vi "Read User Tag.vi"(8 "error in":errorcluster, 11 "MB_TCP session in":refnum<class "MB_Master_TCP.lvclass">) -> (0 "error out":errorcluster, 2 "Value":string, 3 "MB session out":refnum<class "MB_Master_TCP.lvclass">)   [LabVIEW 2024, in "Bronkhorst Flexi-Flow ModbusTCP API.lvlib"]
uses:
  Bronkhorst Flexi-Flow ModbusTCP API.lvlib
  <vilib>/Plasmionique/MB Master/MB_Master_TCP/MB_Master_TCP.lvclass
  PDU Address String Params--ring.ctl
  <vilib>/Utility/error.llb/whitespace.ctl
  <vilib>/Utility/error.llb/Trim Whitespace One-Sided.vi
  Read String Register.vi
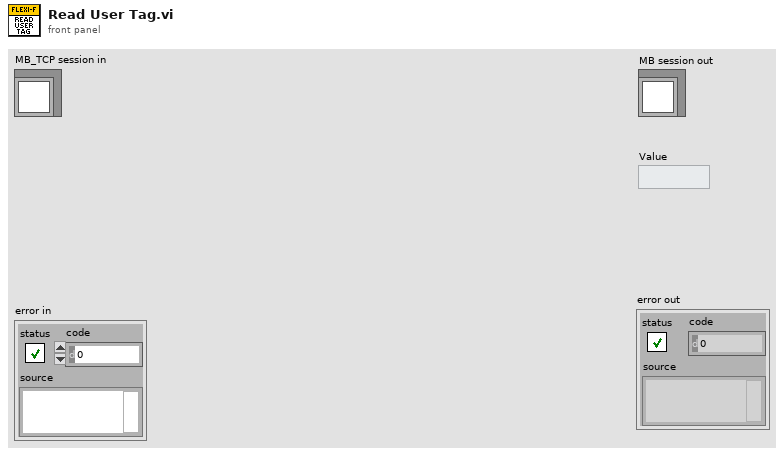
[diagram p1: front panel]
types:
  T1 = typedef "whitespace.ctl" = u16
  T2 = typedef "Bronkhorst Flexi-Flow ModbusTCP API.lvlib/PDU Address String Params--ring.ctl" = u16
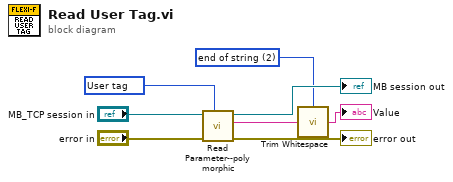
[diagram p0: block diagram]
diagram:
  w1 = T1 2 items=["both", "start of string", "end of string"] ("location (both)")
  w8 = T2 61744 items=["Fluid name"=33160, "Capacity unit"=33272, "User tag"=61744] ("PDU Address String Params")
  n1 = call-poly "Read Parameter--polymorphic.vi"("PDU Address String Params"=w8, "error in"="error in", "MB_TCP session in"="MB_TCP session in") -> ("error out"=→"error out":errorcluster, "Value"=w3:string, "MB session out"=→"MB session out":refnum<class "MB_Master_TCP.lvclass">)  [unwired: 6 in]
  n2 = call <vilib>:"Trim Whitespace.vi"("string"=w3, "location (both)"=w1) -> ("trimmed string"=→"Value":string)
